vi "Loop Init.vi"(8 "error in (no error)":errorcluster) -> (0 "error out":errorcluster, 2 "Action":T1, 3 "Data":variant)   [LabVIEW 2020, in "Controller.lvlib"]
uses:
  Controller.lvlib
  Private Controls/Module Action.ctl
  Private Controls/Element.ctl
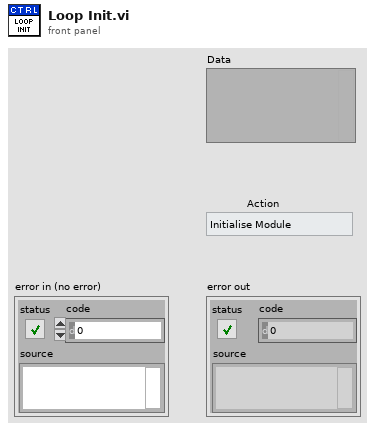
[diagram p1: front panel]
types:
  T1 = typedef "Controller.lvlib/Module Action.ctl" = enum16{"Initialise Module", "Connect", "Setup", "Pause", "Start", "Search Network", "Get Local", "Stop", "Wait: Time Elapsed", "Error", "Exit"}
  T2 = typedef "Controller.lvlib/Element.ctl" = cluster{"Action":T1, "Data":variant}
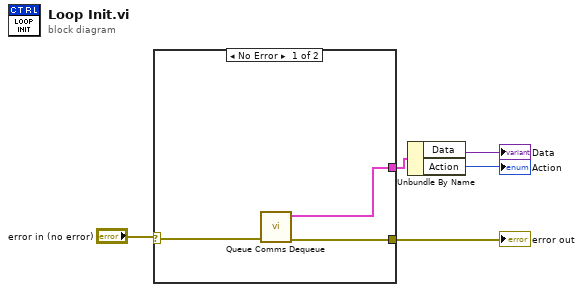
[diagram p0: block diagram]
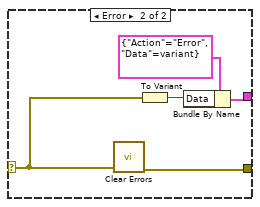
[diagram p2: hidden frame]
diagram:
  n1 = case shown="No Error" "error in (no error)" {
    selector: "error in (no error)" -> [w8 w10]
    tunnel: [w7 w13] -> w4
    tunnel: [w6 w9] -> w3
    frame No Error {
      n2 = call "Queue Comms Dequeue.vi"("error in (no error)"=w8) -> ("error out"=w7:errorcluster, "Element"=w6:T2)  [unwired: 9 in]
    }
    frame Error {
      n3 = call <vilib>:"Clear Errors.vi"("error in (no error)"=w10) -> ("error out"=w13:errorcluster)  [unwired: 5 in, 1 out]
      n4 = To Variant(anything=w10) -> (Variant=w11:variant)
      n5 = Bundle By Name(cluster=T2 {"Action"=enum."Error", "Data"=variant} ("Element"), "Data"=w11) -> (w9:T2)
    }
  }
  "error out" <- w4
  n6 = Unbundle By Name(w3) -> ("Data"=→"Data":variant, "Action"=→"Action":T1)
